vi "命令输出.vi"(8 "error in (no error)":errorcluster caption="错误输入（无错误）", 11 "TimingControl 输入":refnum<class "TimingControl.lvclass">) -> (0 "error out":errorcluster caption="错误输出", 2 "数据":cluster{"启动":bool, "控制命令":T1, "测量参数":T2}, 3 "TimingControl 输出":refnum<class "TimingControl.lvclass">)   [LabVIEW 2022 SP3, in "TimingControl.lvlib" / "TimingControl.lvclass"]
uses:
  TimingControl.lvclass
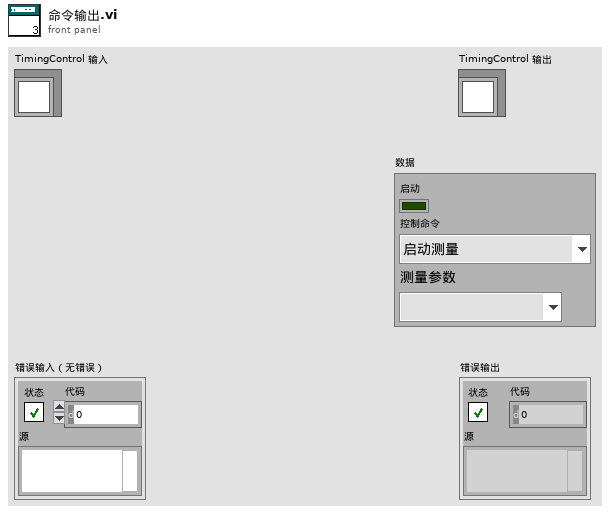
[diagram p1: front panel]
types:
  T1 = typedef "TimingControl.lvlib/TimingControl.lvclass/国标控制命令.ctl" = enum16{"启动测量", "标样核查", "零点核查", "跨度核查", "空白测试", "平行样测试", "加标回收", "空白校准", "标样校准", "初始化（清洗）", "停止测试", "仪器重启", "校时", "模式设置", "测量间隔设置"}
  T2 = typedef "TimingControl.lvlib/TimingControl.lvclass/测量参数.ctl" = u16
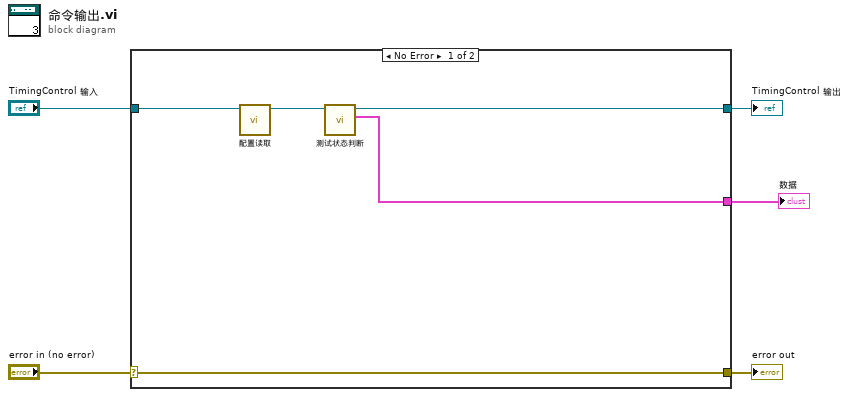
[diagram p0: block diagram]
diagram:
  n1 = case shown="No Error" "error in (no error)" {
    selector: "error in (no error)" -> [w10 w12]
    tunnel: [w10 w12] -> w4
    tunnel: [w7 w11] -> w2
    tunnel: "TimingControl 输入" -> [w6 w11]
    tunnel: [w9 _] -> w1
    frame No Error {
      n2 = call "配置读取.vi"("TimingControl 输入"=w6) -> ("TimingControl 输出"=w8:refnum<class "TimingControl.lvclass">)  [unwired: 9 in, 1 out]
      n3 = call "测试状态判断.vi"("TimingControl 输入"=w8) -> ("数据"=w9:cluster{"启动":bool, "控制命令":T1, "测量参数":T2}, "TimingControl 输出"=w7:refnum<class "TimingControl.lvclass">)  [unwired: 9 in]
    }
    frame Error {
    }
  }
  "error out" <- w4
  "TimingControl 输出" <- w2
  "数据" <- w1
